vi "Page Settings.vi"() -> ()   [LabVIEW 2018, in "Main.lvlib"]
uses:
  Main.lvlib
  Exit/Exit.lvlib
panel:
  in  "Settings Lbx":i32(listbox)=-1 caption="Settings"
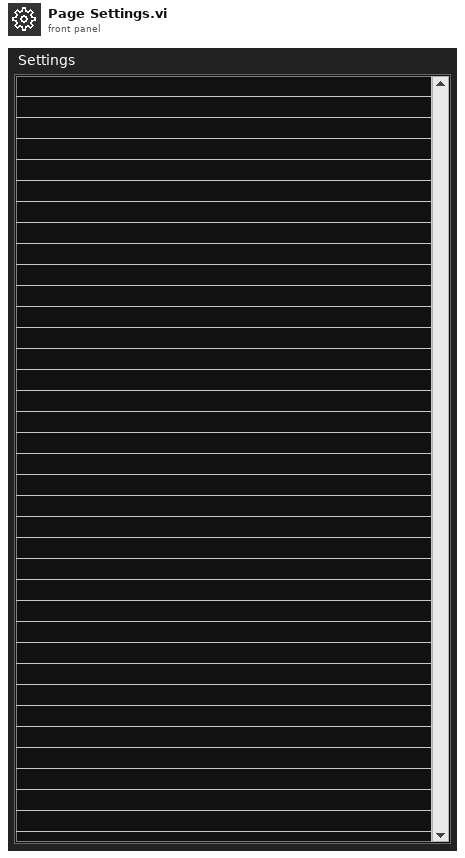
[diagram p1: front panel]
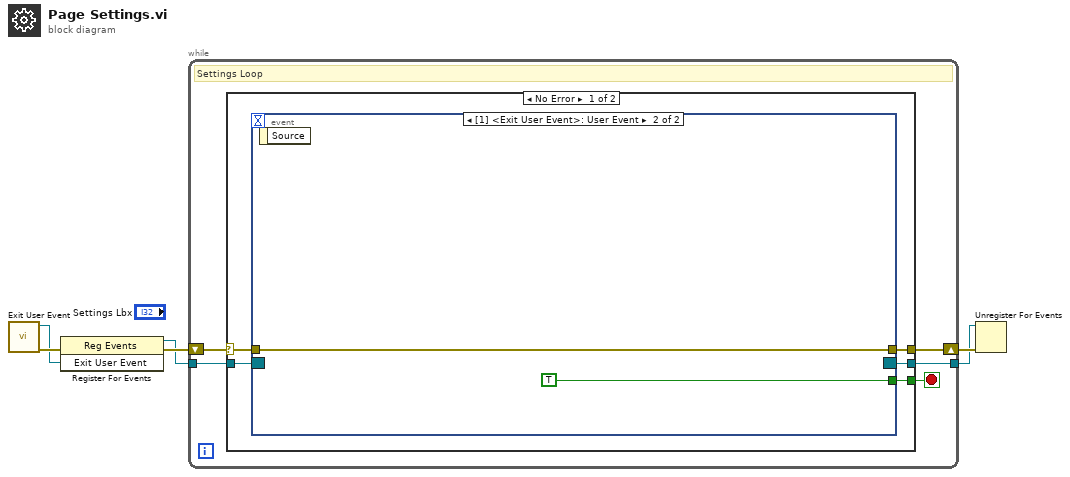
[diagram p0: block diagram]
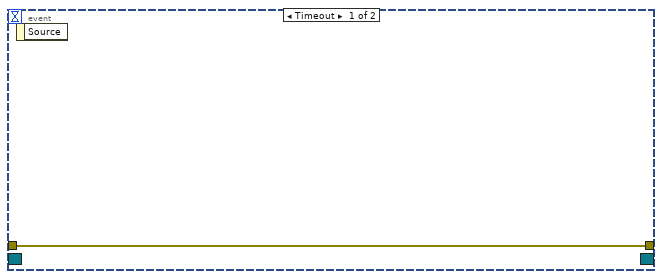
[diagram p2: hidden frame]
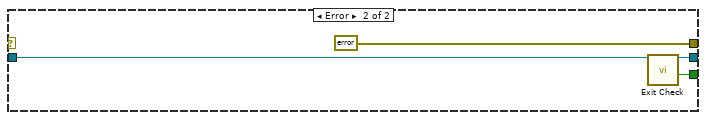
[diagram p3: hidden frame]
diagram:
  n1 = call "Exit User Event.vi"() -> ("error out"=w5:errorcluster, "Exit User Event"=w4:refnum<user-event>)  [unwired: 10 in]
  n2 = register-events(error in=w5, w4) -> (reference out=w3:refnum<event-registration>, error out=w6:errorcluster)  [unwired: 1 in]
  n3 = while {
    tunnel: w3 -> [w10]
    shift-right: [w9] -> w2
    shift-left: w6 -> [w11]
    tunnel: [w7] -> w1
    stop <- w8 stop-if-true
    # "Settings Loop"
    n4 = case shown="No Error" w11 {
      selector: w11 -> [w16 _]
      tunnel: w10 -> [w15 w20]
      tunnel: [w14 errorcluster {"status"=FALSE, "code"=0, "source"=""} ("error IO")] -> w9
      tunnel: [w12 w21] -> w8
      tunnel: [w13 w20] -> w7
      frame No Error {
        n5 = event shown="[1] <Exit User Event>: User Event" {
          selector: w15 -> [_ _]
          dyn-events: [_ _] -> w13
          timeout: _ -> [_ _]
          tunnel: w16 -> [w17 w19]
          tunnel: [w17 w19] -> w14
          tunnel: [_ TRUE] -> w12
          event Timeout {
            n6 = event-data() -> ()  [unwired: 1 in, 1 out]
          }
          event User Event {
            n7 = event-data() -> ()  [unwired: 1 in, 1 out]
          }
        }
      }
      frame Error {
        n8 = call "Exit Check.vi"() -> ("Exit?"=w21:bool)  [unwired: 10 in, 1 out]
      }
    }
  }
  n9 = Unregister For Events(event registration refnum=w1, error in=w2) -> ()  [unwired: 1 out]
